vi "Initialize.vi"(8 "error in":errorcluster, 9 "parameters":variant, 10 "path":path, 11 "repository in":refnum<class "database file.lvclass">) -> (0 "error out":errorcluster, 3 "repository out":refnum<class "database file.lvclass">)   [LabVIEW 2013, in "database file.lvclass"]
doc: "Initializes the repo. StoreClassPath method should be called in this VI"
uses:
  database file.lvclass
  J1939 Library/Configuration/TypeDefs/J1939 db.ctl
  J1939 Library/Configuration/TypeDefs/J1939 db frame.ctl
  J1939 Library/Configuration/TypeDefs/J1939 db signal.ctl
  database file.lvclass/database file.ctl
  <vilib>/NI/Configuration Framework/Repository/NISE_CEF_Repository.lvclass
  J1939FullDB.vi
  J1939 Library/J1939.lvlib
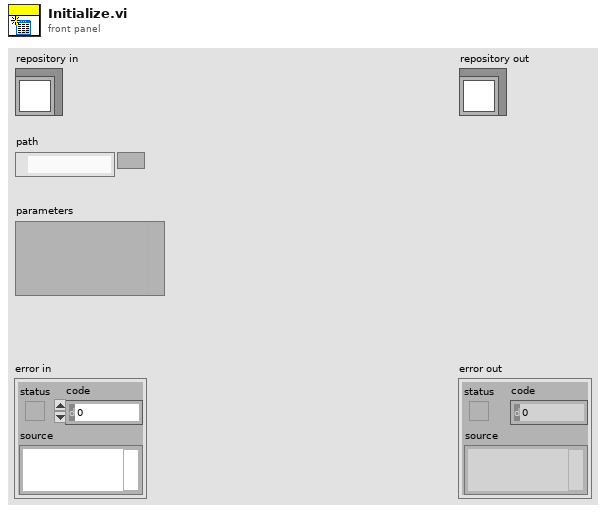
[diagram p1: front panel]
types:
  T1 = typedef "J1939.lvlib/J1939 db.ctl" = cluster{"BaudRate":u32, "CAN.IoMode":u32, "J1939 Network Address":u8, "Name":u64, "frames":T2[]}
  T2 = typedef "J1939.lvlib/J1939 db frame.ctl" = cluster{"name":string, "Priority":u8, "PGN":u32, "Reserved Bit":u8, "Data page":u8, "PDU Format":u8, "PDU Specific":u8, "Source Address":u8, "PayldLen":u32, "signals":T3[], "Comment":string, "can timing type":u32, "transmit time":dbl, "direction":u16}
  T3 = typedef "J1939.lvlib/J1939 db signal.ctl" = cluster{"NameShort":string, "SPN":i32, "StartBit":u32, "NumBits":u32, "DataType":u32, "ByteOrdr":u32, "ScaleFac":dbl, "ScaleOff":dbl, "Max":dbl, "Min":dbl, "Default":dbl, "Unit":string, "Comment":string}
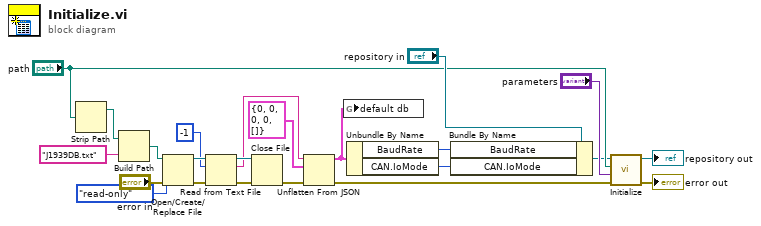
[diagram p0: block diagram]
diagram:
  n1 = Strip Path(path="path") -> (stripped path=w18:path)  [unwired: 1 out]
  n2 = Build Path(base path=w18, name or relative path="J1939DB.txt") -> (appended path=w16:path)
  n3 = Open/Create/Replace File(file path (use dialog)=w16, error in="error in", access (0:read/write)=enum16{"read/write", "read-only", "write-only"}."read-only") -> (refnum out=w15:refnum<file>, error out=w12:errorcluster)  [unwired: 3 in, 1 out]
  n4 = Read from Text File(file (use dialog)=w15, count=-1, error in=w12) -> (refnum out=w14:refnum<file>, text=w6:string, error out=w11:errorcluster)  [unwired: 1 in, 1 out]
  n5 = Close File(refnum=w14, error in=w11) -> (error out=w10:errorcluster)  [unwired: 1 out]
  n6 = Unflatten From JSON(JSON string=w6, type and defaults=T1 {"BaudRate"=0, "CAN.IoMode"=0, "J1939 Network Address"=0, "Name"=0, "frames"=[]} ("database"), error in (no error)=w10) -> (value=w4:T1, error out=w8:errorcluster)  [unwired: 4 in]
  n7 = global write "J1939FullDB.vi" "default db"(w4) -> ()
  n8 = Unbundle By Name(w4) -> ("BaudRate"=w2:u32, "CAN.IoMode"=w3:u32)
  n9 = Bundle By Name(cluster="repository in", "BaudRate"=w2, "CAN.IoMode"=w3) -> (w9:refnum<class "database file.lvclass">)
  n10 = call-parent "Initialize.vi"("error in"=w8, "parameters"="parameters", "path"="path", "repository in"=w9) -> ("error out"=→"error out":errorcluster, "repository out"=→"repository out":refnum<class "database file.lvclass">)  [unwired: 6 in]
